vi "JSON to Variant.vi"(8 "error in (no error)":errorcluster, 10 "Variant (Data Type)":variant, 11 "JSON Value":refnum<class "JSON Value.lvclass">) -> (0 "error out":errorcluster, 2 "Variant out":variant)   [LabVIEW 2011, in "Variant JSON.lvlib"]
doc: "Converts a JSON value object into a LabVIEW datatype.\n\nElements in the <b>Variant (Data Type)</b> are used to retrieve information from <b>JSON Value</b>.\n\nCopyright 2012 James David Powell, Shaun Rumbell and Ton Plomp\nMore information on http://lavag.org/topic/16217-cr-json-labview"
uses:
  Variant JSON.lvlib
  JSON Value/JSON Value.lvclass
  JSON Object/JSON Object.lvclass
  JSON Value/Get as JSON string.vi
  JSON Scalar/Get as I32.vi
  JSON Scalar/Get as I64.vi
  JSON Scalar/Get as U32.vi
  JSON Scalar/Get as U64.vi
  JSON Scalar/Get as SGL.vi
  JSON Scalar/Get as DBL.vi
  JSON Scalar/Get as EXT.vi
  JSON Scalar/Get as Boolean.vi
  JSON Value/Get Item by name array.vi
  JSON Scalar/Get as Path.vi
  <userlib>/_OpenG.lib/array/array.llb/Conditional Auto-Indexing Tunnel (String)__ogtk.vi
  JSON Scalar/Get as Timestamp.vi
  JSON Scalar/JSON Scalar.lvclass
  Get Polymorphic/JSON GetSet.lvlib
  <vilib>/Utility/VariantDataType/VariantType.lvlib
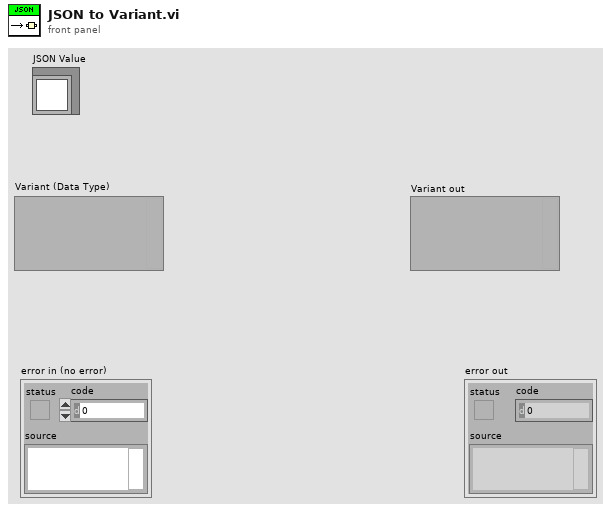
[diagram p1: front panel]
types:
  T1 = typedef "VariantType.lvlib/Type.ctl" = enum8{"Invalid Type", "Void", "I8", "I16", "I32", "I64", "U8", "U16", "U32", "U64", "Single Float", "Double Float", "Extended Float", "Single Complex", "Double Complex", "Extended Complex", "Enum U8", "Enum U16", "Enum U32", "Enum U64", "Single Float With Unit", "Double Float With Unit", "Extended Float With Unit", "Single Complex with Unit", "Double Complex with Unit", "Extended Complex with Unit", "Boolean", "String", "Path", "Picture", "Tag", "Array", "Cluster", "Variant", "LV Variant", "Waveform", "Timestamp", "Digital Waveform", "Digital Data", "ExpressData", "Refnum", "External Data", "VI", "Poly VI", "LabVIEW Class Instance", "Fixed Point"}
  T2 = typedef "JSON Scalar.lvclass/Variant Data Typdef.ctl" = cluster{"Type Enum":T1, "Name":string, "Variant":variant}
  T3 = cluster{"empty?":bool, "code":i32, "source":string}
  T4 = typedef "VariantType.lvlib/RefnumType.ctl" = enum16{"NotARefnum", "UnknownRefnum", "Generic", "Datalog", "ByteStream", "Device", "Occurence", "TCPNetConnection", "Auto", "Menu", "Imaq", "Hardware", "DataSocket", "Visa", "IVI", "UDPNetConnection", "Notifier", "Queue", "Irda", "EventReg", "DotNet", "UserEvent", "Callback", "UNUSED_EMPTY_POSITION", "BlueToothNetConnection", "LVObjApp", "LVObjVI", "LVObjUnknown", "GenericClass", "UserDefinedRefnumTag", "DataValue"}
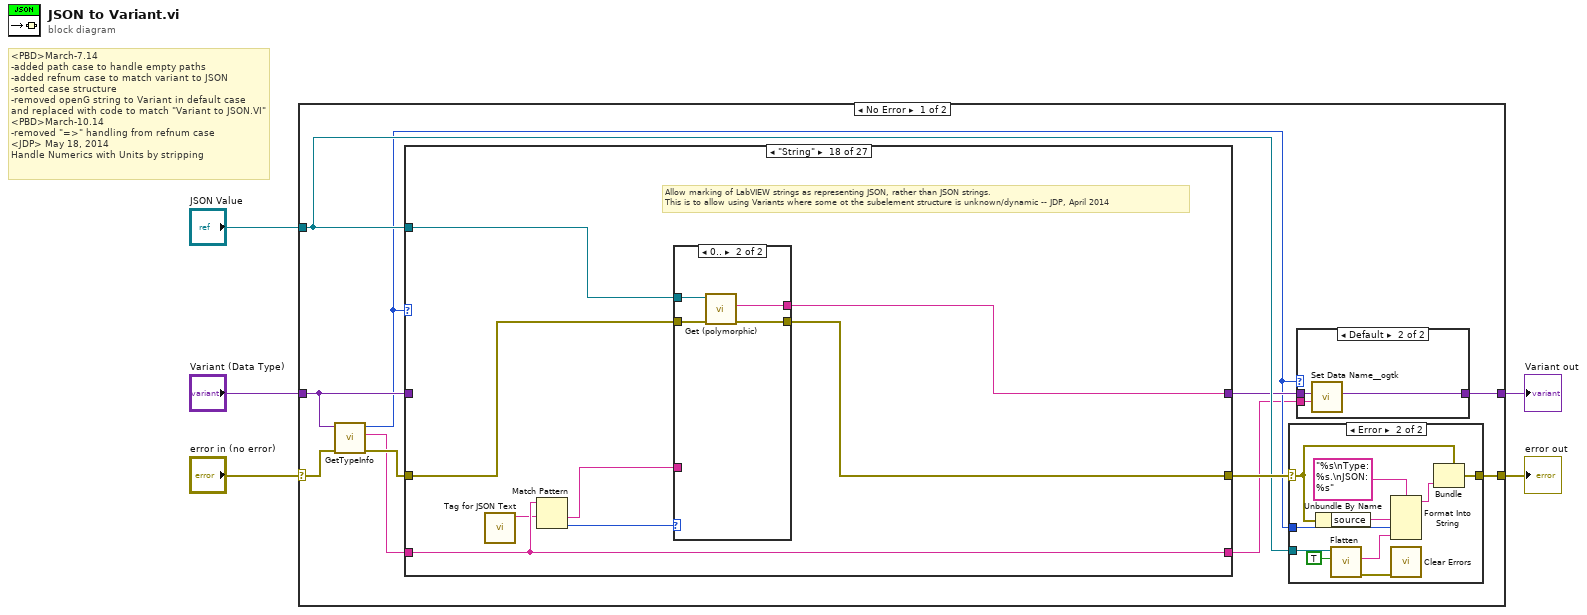
[diagram p0: block diagram]
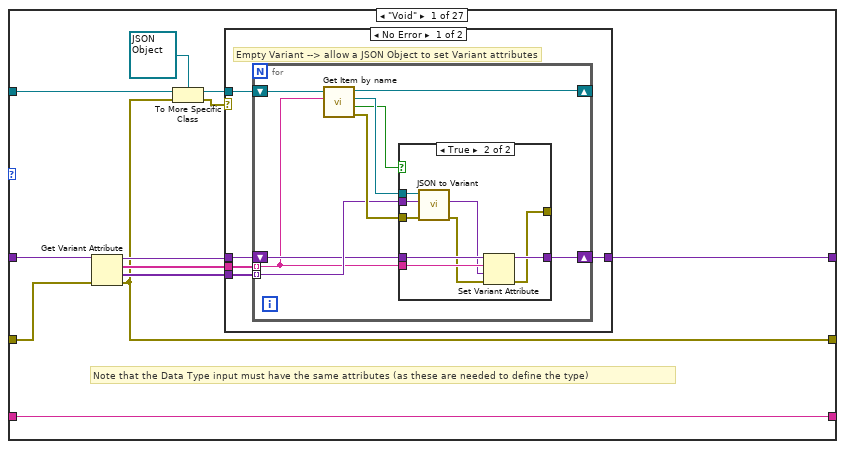
[diagram p4: hidden frame]
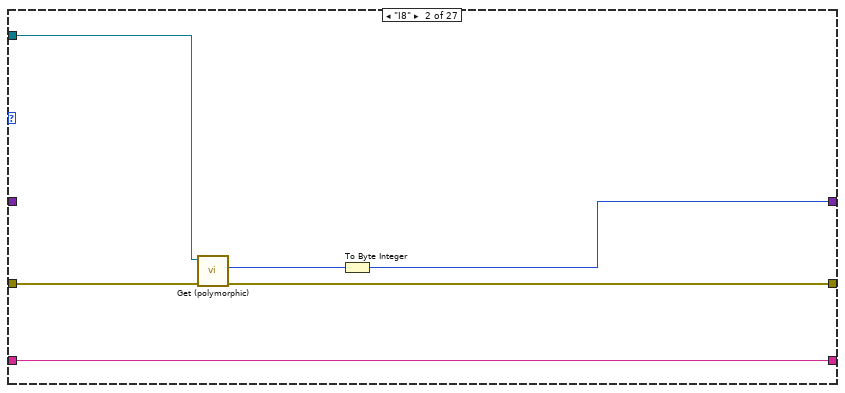
[diagram p7: hidden frame]
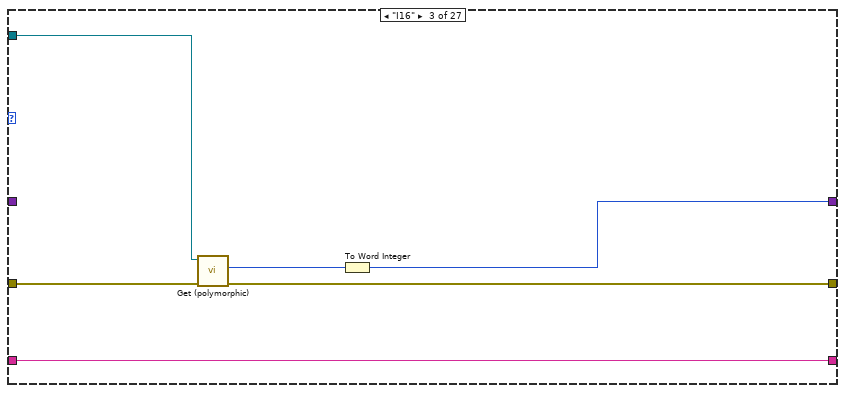
[diagram p8: hidden frame]
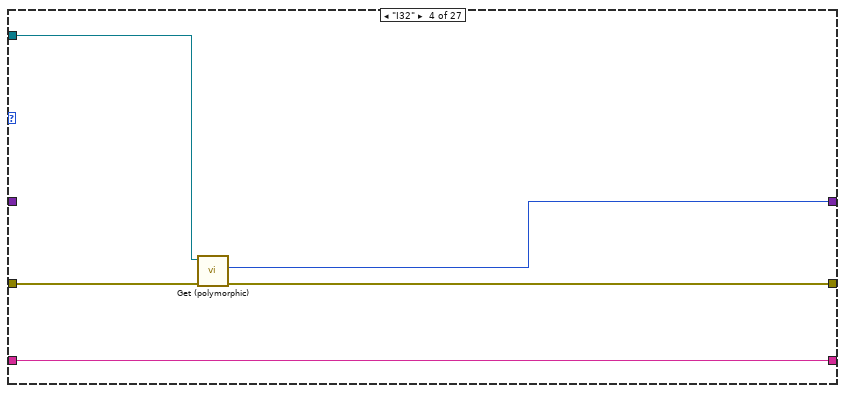
[diagram p9: hidden frame]
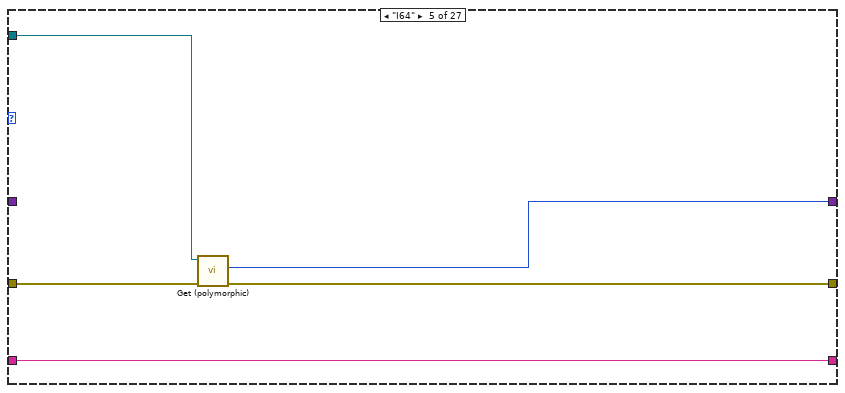
[diagram p10: hidden frame]
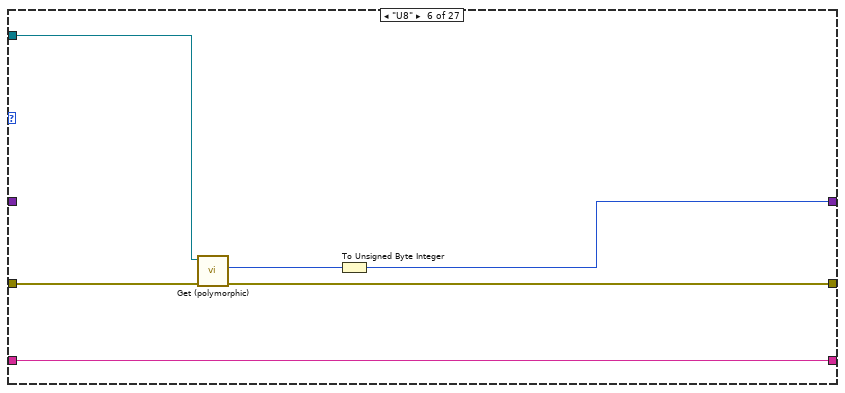
[diagram p11: hidden frame]
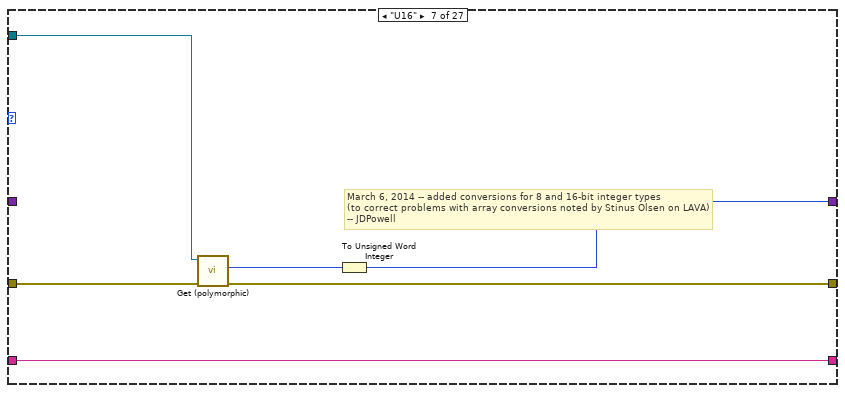
[diagram p12: hidden frame]
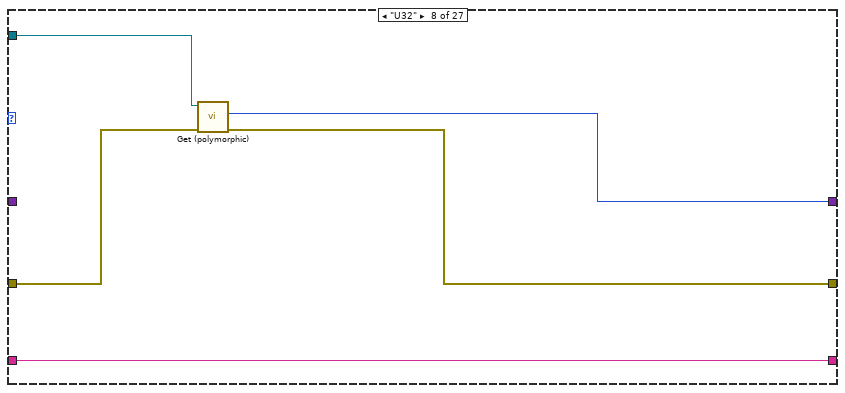
[diagram p13: hidden frame]
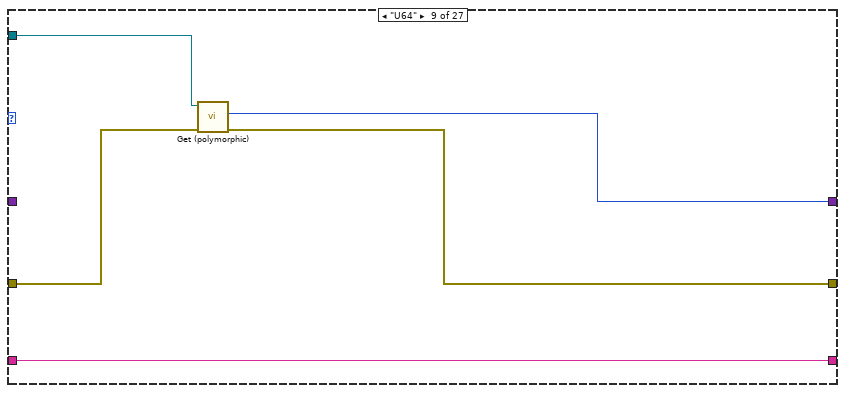
[diagram p14: hidden frame]
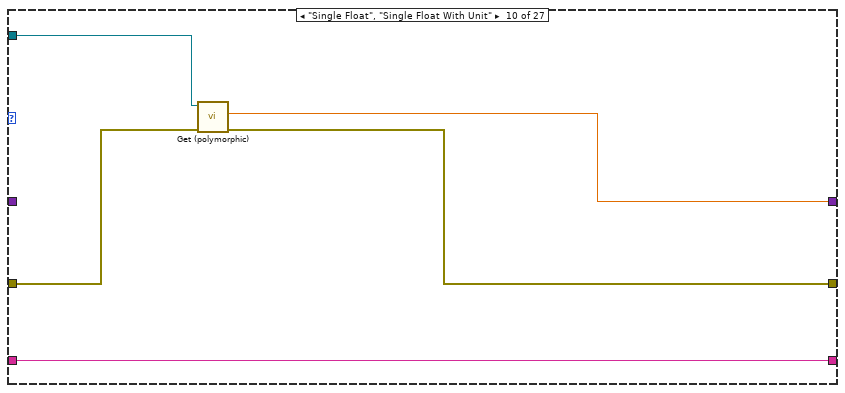
[diagram p15: hidden frame]
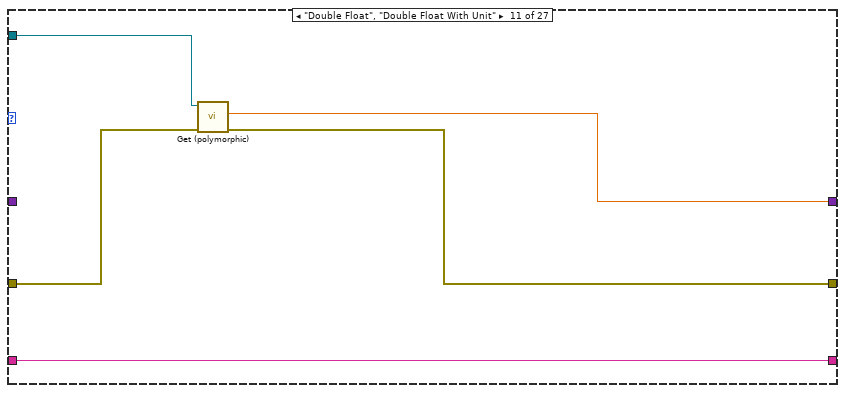
[diagram p16: hidden frame]
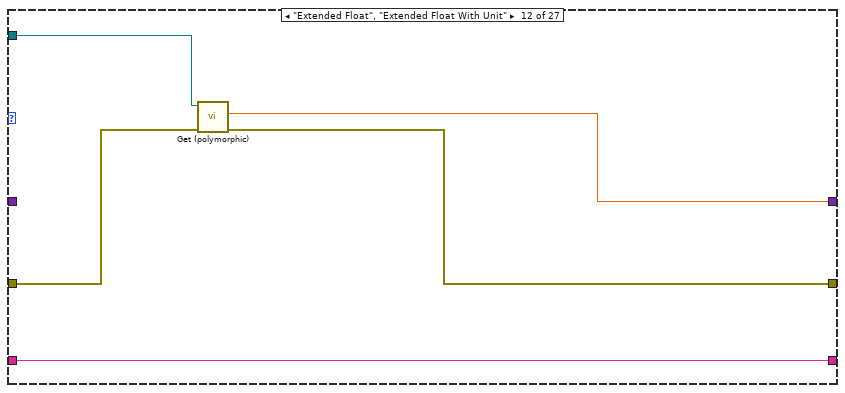
[diagram p17: hidden frame]
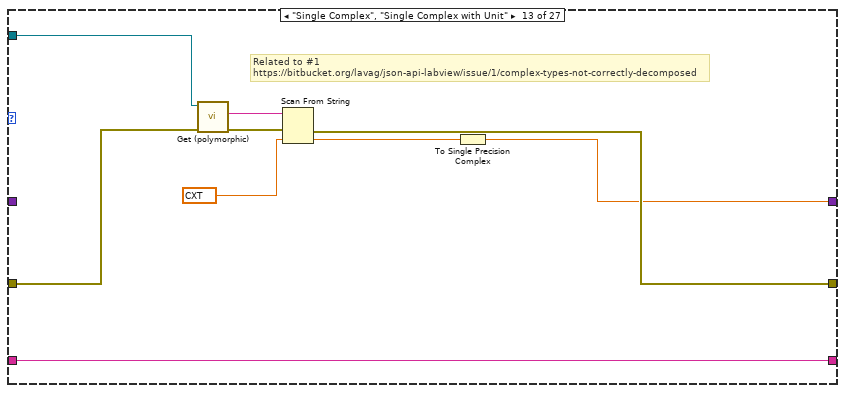
[diagram p18: hidden frame]
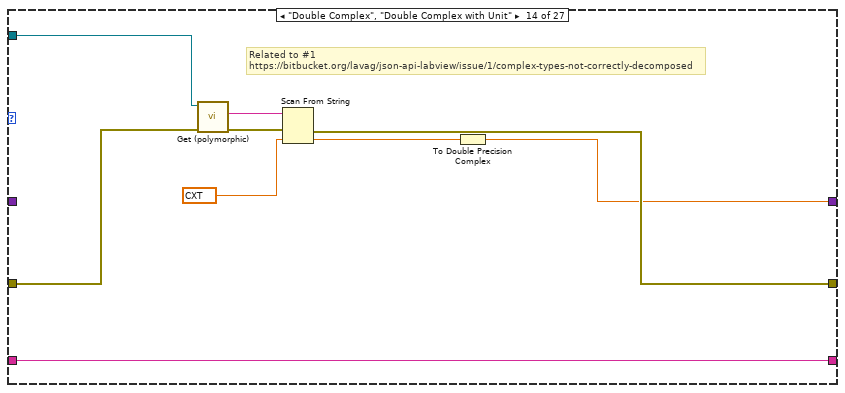
[diagram p19: hidden frame]
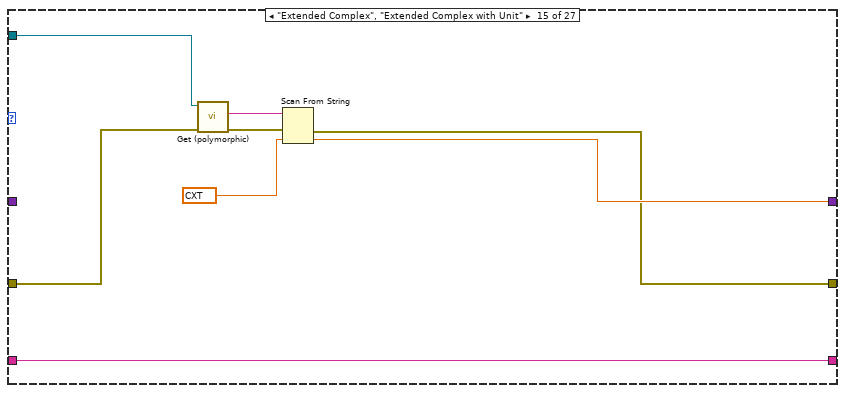
[diagram p20: hidden frame]
diagram:
  # "<PBD>March-7.14\n-added path case to handle empty paths\n-added refnum case to match variant to JSON\n-sorted case structure\n-removed openG string to Variant in default case \nand replaced with code to match \"Variant to JSON.VI\"\n<PBD>March-10.14\n-removed \"=>\" handling from refnum case\n<JDP> May 18, 2014\nHandle Numerics with Units by stripping"
  n1 = case shown="No Error" "error in (no error)" {
    selector: "error in (no error)" -> [w10 w326]
    tunnel: [w15 w326] -> w4
    tunnel: "Variant (Data Type)" -> [w11 w325]
    tunnel: "JSON Value" -> [w14 _]
    tunnel: [w12 w325] -> w1
    frame No Error {
      n2 = call <vilib>:"GetTypeInfo.vi"("error in (no error)"=w10, "Variant"=w11) -> ("error out"=w9:errorcluster, "Name"=w7:string, "Type Enum"=w8:T1)  [unwired: 5 in, 2 out]
      n3 = case shown="\"String\"" w8 {
        tunnel: w11 -> [w39 _ _ _ _ _ _ _ _ _ _ _ _ _ _ w162 _ _ _ w191 w199 w244 _ _ w262 w292 w321]
        tunnel: w9 -> [w34 w73 w79 w84 w89 w95 w101 w106 w111 w116 w121 w126 w136 w145 w153 w157 w165 w173 w187 w193 w198 w243 w249 w253 w261 _ w324]
        tunnel: [w33 w72 w78 w83 w88 w94 w100 w105 w110 w115 w120 w125 w131 w140 w148 w156 w164 w172 w186 w192 w205 w246 w248 w254 w258 w293 w319] -> w16
        tunnel: w14 -> [w43 w75 w81 w86 w91 w97 w103 w108 w113 w118 w123 w128 w137 w146 w154 w160 w167 w175 w188 w194 w203 w245 w251 w256 w260 w295 w323]
        tunnel: [w35 w71 w77 w85 w90 w93 w99 w107 w112 w117 w122 w127 w130 w139 w150 w161 w166 w174 w185 w189 w201 w238 w250 w255 w259 w294 w318] -> w13
        tunnel: w7 -> [w32 w70 w76 w82 w87 w92 w98 w104 w109 w114 w119 w124 w129 w138 w147 w155 w163 w171 w184 w190 w195 w237 w247 w252 w257 w301 w316]
        tunnel: [w32 w70 w76 w82 w87 w92 w98 w104 w109 w114 w119 w124 w129 w138 w147 w155 w163 w171 w184 w190 w195 w237 w247 w252 w257 w301 w316] -> w6
        frame "Void" {
          # "Note that the Data Type input must have the same attributes (as these are needed to define the type)"
          n4 = Get Variant Attribute(Variant=w39, error in=w34) -> (duplicate Variant=w38:variant, names=w37:string[], values=w36:variant[], error out=w33:errorcluster)  [unwired: 2 in]
          n5 = To More Specific Class(target class=refnum<class "JSON Object.lvclass"> refnum ("JSON Object in"), reference=w43, error in=w33) -> (specific class reference=w41:refnum<class "JSON Object.lvclass">, error out=w40:errorcluster)
          n6 = case shown="No Error" w40 {
            tunnel: w41 -> [w45 _]
            tunnel: w38 -> [w46 w69]
            tunnel: w37 -> [w48 _]
            tunnel: w36 -> [w47 _]
            tunnel: [w44 w69] -> w35
            frame No Error {
              # "Empty Variant --> allow a JSON Object to set Variant attributes"
              n7 = for {
                tunnel: w48 -> [w51] mode=indexing
                tunnel: w47 -> [w53] mode=indexing
                shift-right: [w50] -> w44
                shift-left: w46 -> [w52]
                shift-right: [w49] -> _
                shift-left: w45 -> [w54]
                n8 = call-dynamic "Get Item by name.vi"("name"=w51, "JSON Object in"=w54) -> ("error out"=w57:errorcluster, "found"=w55:bool, "Value"=w56:refnum<class "JSON Value.lvclass">, "JSON Object out"=w49:refnum<class "JSON Object.lvclass">)  [unwired: 6 in]
                n9 = case shown="True" w55 {
                  tunnel: w57 -> [w59 w68]
                  tunnel: [w59 w60] -> _
                  tunnel: w53 -> [_ w67]
                  tunnel: w56 -> [_ w66]
                  tunnel: w52 -> [w58 w65]
                  tunnel: w51 -> [_ w64]
                  tunnel: [w58 w63] -> w50
                  frame False {
                  }
                  frame True {
                    n10 = call "JSON to Variant.vi"("error in (no error)"=w68, "Variant (Data Type)"=w67, "JSON Value"=w66) -> ("error out"=w61:errorcluster, "Variant out"=w62:variant)  [unwired: 7 in]
                    n11 = Set Variant Attribute(Variant=w65, name=w64, value=w62, error in=w61) -> (Variant out=w63:variant, error out=w60:errorcluster)  [unwired: 1 out]
                  }
                }
              }
            }
            frame Error {
            }
          }
        }
        frame "I8" {
          n12 = call-poly "Get (polymorphic).vi"("error in (no error)"=w73, "JSON Scalar in"=w75) -> ("error out"=w72:errorcluster, "Number"=w74:i32)  [unwired: 7 in, 1 out]
          n13 = To Byte Integer(number=w74) -> (8bit integer=w71:i8)
        }
        frame "I16" {
          n14 = call-poly "Get (polymorphic).vi"("error in (no error)"=w79, "JSON Scalar in"=w81) -> ("error out"=w78:errorcluster, "Number"=w80:i32)  [unwired: 7 in, 1 out]
          n15 = To Word Integer(number=w80) -> (16bit integer=w77:i16)
        }
        frame "I32" {
          n16 = call-poly "Get (polymorphic).vi"("error in (no error)"=w84, "JSON Scalar in"=w86) -> ("error out"=w83:errorcluster, "Number"=w85:i32)  [unwired: 7 in, 1 out]
        }
        frame "I64" {
          n17 = call-poly "Get (polymorphic).vi"("error in (no error)"=w89, "JSON Scalar in"=w91) -> ("error out"=w88:errorcluster, "Number"=w90:i64)  [unwired: 7 in, 1 out]
        }
        frame "U8" {
          n18 = call-poly "Get (polymorphic).vi"("error in (no error)"=w95, "JSON Scalar in"=w97) -> ("error out"=w94:errorcluster, "Number"=w96:u32)  [unwired: 7 in, 1 out]
          n19 = To Unsigned Byte Integer(number=w96) -> (unsigned 8bit integer=w93:u8)
        }
        frame "U16" {
          # "March 6, 2014 -- added conversions for 8 and 16-bit integer types\n(to correct problems with array conversions noted by Stinus Olsen on LAVA)\n-- JDPowell"
          n20 = call-poly "Get (polymorphic).vi"("error in (no error)"=w101, "JSON Scalar in"=w103) -> ("error out"=w100:errorcluster, "Number"=w102:u32)  [unwired: 7 in, 1 out]
          n21 = To Unsigned Word Integer(number=w102) -> (unsigned 16bit integer=w99:u16)
        }
        frame "U32" {
          n22 = call-poly "Get (polymorphic).vi"("error in (no error)"=w106, "JSON Scalar in"=w108) -> ("error out"=w105:errorcluster, "Number"=w107:u32)  [unwired: 7 in, 1 out]
        }
        frame "U64" {
          n23 = call-poly "Get (polymorphic).vi"("error in (no error)"=w111, "JSON Scalar in"=w113) -> ("error out"=w110:errorcluster, "Number"=w112:u64)  [unwired: 7 in, 1 out]
        }
        frame "Single Float", "Single Float With Unit" {
          n24 = call-poly "Get (polymorphic).vi"("error in (no error)"=w116, "JSON Value in"=w118) -> ("error out"=w115:errorcluster, "Number"=w117:sgl)  [unwired: 7 in, 1 out]
        }
        frame "Double Float", "Double Float With Unit" {
          n25 = call-poly "Get (polymorphic).vi"("error in (no error)"=w121, "JSON Value in"=w123) -> ("error out"=w120:errorcluster, "Number"=w122:dbl)  [unwired: 7 in, 1 out]
        }
        frame "Extended Float", "Extended Float With Unit" {
          n26 = call-poly "Get (polymorphic).vi"("error in (no error)"=w126, "JSON Value in"=w128) -> ("error out"=w125:errorcluster, "Number"=w127:ext)  [unwired: 7 in, 1 out]
        }
        frame "Single Complex", "Single Complex with Unit" {
          # "Related to #1\nhttps://bitbucket.org/lavag/json-api-labview/issue/1/complex-types-not-correctly-decomposed"
          n27 = call-poly "Get (polymorphic).vi"("error in (no error)"=w136, "JSON Scalar in"=w137) -> ("error out"=w132:errorcluster, "LabVIEW Text"=w135:string)  [unwired: 7 in, 1 out]
          n28 = Scan From String(input string=w135, error in=w132, default 1=cxt 0.0+0.0i) -> (error out=w131:errorcluster, output 1=w133:cxt)  [unwired: 2 in, 2 out]
          n29 = To Single Precision Complex(1:w133) -> (0:w130:csg)
        }
        frame "Double Complex", "Double Complex with Unit" {
          # "Related to #1\nhttps://bitbucket.org/lavag/json-api-labview/issue/1/complex-types-not-correctly-decomposed"
          n30 = call-poly "Get (polymorphic).vi"("error in (no error)"=w145, "JSON Scalar in"=w146) -> ("error out"=w141:errorcluster, "LabVIEW Text"=w144:string)  [unwired: 7 in, 1 out]
          n31 = Scan From String(input string=w144, error in=w141, default 1=cxt 0.0+0.0i) -> (error out=w140:errorcluster, output 1=w142:cxt)  [unwired: 2 in, 2 out]
          n32 = To Double Precision Complex(1:w142) -> (0:w139:cdb)
        }
        frame "Extended Complex", "Extended Complex with Unit" {
          n33 = call-poly "Get (polymorphic).vi"("error in (no error)"=w153, "JSON Scalar in"=w154) -> ("error out"=w149:errorcluster, "LabVIEW Text"=w152:string)  [unwired: 7 in, 1 out]
          n34 = Scan From String(input string=w152, error in=w149, default 1=cxt 0.0+0.0i) -> (error out=w148:errorcluster, output 1=w150:cxt)  [unwired: 2 in, 2 out]
        }
        frame "Enum U8".."Enum U64" {
          n35 = call-poly "Get (polymorphic).vi"("error in (no error)"=w157, "JSON Scalar in"=w160) -> ("error out"=w158:errorcluster, "LabVIEW Text"=w159:string)  [unwired: 7 in, 1 out]
          n36 = call <userlib>:"Set Enum String Value__ogtk.vi"("error in (no error)"=w158, "String Value"=w159, "Default Enum Value"=w162) -> ("error out"=w156:errorcluster, "Enum"=w161:variant)  [unwired: 7 in]
        }
        frame "Boolean" {
          n37 = call-poly "Get (polymorphic).vi"("error in (no error)"=w165, "JSON Value in"=w167) -> ("error out"=w164:errorcluster, "Boolean"=w166:bool)  [unwired: 7 in, 1 out]
        }
        frame "String" {
          # "Allow marking of LabVIEW strings as representing JSON, rather than JSON strings.\nThis is to allow using Variants where some ot the subelement structure is unknown/dynamic -- JDP, April 2014"
          n38 = call "Tag for JSON Text.vi"() -> ("Tag for JSON text"=w168:string)  [unwired: 11 in]
          n39 = Match Pattern(string=w171, regular expression=w168) -> (after substring=w170:string, offset past match=w169:i32)  [unwired: 1 in, 2 out]
          n40 = case shown="0.." w169 {
            tunnel: w175 -> [w179 w183]
            tunnel: [w178 w182] -> w174
            tunnel: w173 -> [w177 w181]
            tunnel: [w176 w180] -> w172
            tunnel: w170 -> [_ _]
            frame ..-1 {
              n41 = call-poly "Get (polymorphic).vi"("error in (no error)"=w177, "JSON Scalar in"=w179) -> ("error out"=w176:errorcluster, "LabVIEW Text"=w178:string)  [unwired: 7 in, 1 out]
            }
            frame 0.. {
              n42 = call-poly "Get (polymorphic).vi"("error in (no error)"=w181, "JSON Value in"=w183) -> ("error out"=w180:errorcluster, "String"=w182:string)  [unwired: 8 in]
            }
          }
        }
        frame "Path" {
          n43 = call-poly "Get (polymorphic).vi"("error in (no error)"=w187, "JSON Scalar in"=w188) -> ("error out"=w186:errorcluster, "path"=w185:path)  [unwired: 7 in, 1 out]
        }
        frame "Array" {
          # "Dec 2015, JDP rewrite for higher speed with large arrays"
          n44 = call "Get Array as Variant.vi"("error in (no error)"=w193, "Variant (Data Type)"=w191, "JSON Value in"=w194) -> ("error out"=w192:errorcluster, "Default VData"=w189:variant)  [unwired: 7 in]
        }
        frame "Cluster" {
          w204 = 91 items=["No error", "Argument error", "Memory is full", "Out of zone", "End of file", "File already open", "Generic file I/O error", "File not found", "File permission error", "Disk is full", "Duplicate path", "Too many files open", "System feature not enabled", "Resource file not found", "Cannot add resource", "Resource not found", "Image not found", "Image memory error", "Pen does not exist", "Config type invalid", "Config token not found", "Config parse error", "Config memory error", "Bad external code format", "Bad external code offset", "External code not present", "Null window", "Destroy window error", "Null menu", "Print aborted", "Bad print record", "Print driver error", "Windows error during printing", "Memory error during printing", "Print dialog error", "Generic print error", "Invalid device refnum", "Device not found", "Device parameter error", "Device unit error", "Cannot open device", "Device call aborted", "Generic error", "Cancelled by user", "Object ID too low", "Object ID too high", "Object not in heap", "Unknown heap", "Unknown object (invalid DefProc)", "Unknown object (DefProc not in table)", "Message out of range", "Invalid (null) method", "Unknown message", "Manager call not supported", "Bad address", "Network operation in progress", "Network operation timed out", "Connection is busy", "Network attribute not supported", "Network error", "Address in use", "System out of memory", "Connection aborted", "Connection refused", "Not connected", "Already connected", "Connection closed", "Initialization error (interapplication manager)", "Bad occurrence", "Wait on unbound occurrence handler", "Occurrence queue overflow", "Datalog type conflict", "Unused", "Unrecognized type (interapplication manager)", "Memory corrupt", "Failed to make temporary DLL", "Old CIN version", "Drag socket not found", "Failed to load drop-object", "Failed to register OLE object", "Failed to release OLE object", "Format specifier type mismatch", "Unknown format specifier", "Too few format specifiers", "Too many format specifiers", "Scan failed", "Newer CIN version", "Error converting to variant", "Runtime menu error", "Password tampered", "Variant attribute not found", "Incompatible variant data type", "Event data is not available", "Event Store is not present", "Occurrence is not found", "Event Queue is not created", "Event info is not available", "Refnum passed is NULL", "Error retrieving Class GUID", "Error retrieving CoClass GUID", "Error retrieving TypeLib GUID.", "Bad built application magic bytes.", "Specific driver is different from the specific driver associated with the Logical Name.", "There is no session opened to the class driver.", "Max Error", "MAX - Error with config objects", "MAX - Error loading configuration", "MAX - Group not supported"]
          # "If an elements fails, set a warning (91)\nIncluding the source JSON string."
          # "<ToDo>\nGo over this error logic"
          # "Throw warning,\nnot an error."
          n45 = call "Variant Decode.vi"("error in (no error)"=w198, "variant"=w199) -> ("error out"=w196:errorcluster, "Variant Data"=w197:T2[])  [unwired: 7 in, 1 out]
          n46 = for {
            shift-right: [w228] -> _
            shift-left: w203 -> [w229]
            tunnel: [w225] -> w202 mode=indexing
            tunnel: [w227] -> w217 mode=indexing
            tunnel: [w221] -> w216 mode=indexing
            tunnel: w197 -> [w224] mode=indexing
            n47 = call "Handle JSON Text Tag.vi"("Variant Data"=w224) -> ("Variant Data (tag stripped)"=w223:T2)  [unwired: 9 in, 1 out]
            n48 = Unbundle By Name(w223) -> ("Name"=w221:string, "Variant"=w222:variant)
            n49 = call-dynamic "Get Item by name.vi"("name"=w221, "JSON Value In"=w229) -> ("error out"=w220:errorcluster, "found"=w218:bool, "Value"=w219:refnum<class "JSON Value.lvclass">, "JSON Value Out"=w228:refnum<class "JSON Value.lvclass">)  [unwired: 6 in]
            n50 = case shown="True" w218 {
              tunnel: w220 -> [w230 w236]
              tunnel: [w230 w235] -> w226
              tunnel: w222 -> [w231 w234]
              tunnel: w219 -> [_ w233]
              tunnel: [w231 w232] -> w225
              frame False {
              }
              frame True {
                n51 = call "JSON to Variant.vi"("error in (no error)"=w236, "Variant (Data Type)"=w234, "JSON Value"=w233) -> ("error out"=w235:errorcluster, "Variant out"=w232:variant)  [unwired: 7 in]
              }
            }
            n52 = Unbundle By Name(w226) -> ("status"=w227:bool)
          }
          n53 = call <userlib>:"Array of VData to VCluster__ogtk.vi"("error in (no error)"=w196, "Array"=w202) -> ("error out"=w200:errorcluster, "VCluster"=w201:variant)  [unwired: 8 in]
          n54 = call-poly <userlib>:"Conditional Auto-Indexing Tunnel__ogtk.vi"("Array in"=w216, "Elements to keep"=w217) -> ("Filtered Array out"=w211:string[])  [unwired: 5 in]
          n55 = Array To Spreadsheet String(delimiter (Tab)="\r\n", array=w211, 3:"%s" ("format string")) -> (spreadsheet string=w212:string)
          n56 = Empty Array?(array=w211) -> (empty?=w208:bool)
          n57 = Format Into String(format string="Failed elements:\n%s", w212) -> (resulting string=w207:string)  [unwired: 2 in, 1 out]
          n58 = Bundle("empty?"=w208, w204, w207) -> (w209:cluster{"empty?":bool, i32, string})  [unwired: 1 in]
          n59 = Select(t=errorcluster {"status"=FALSE, "code"=0, "source"=""} ("error out"), s=w208, f=w209) -> (s? t:f=w206:T3)
          n60 = Merge Errors(w200, w206) -> (w205:errorcluster)
        }
        frame "Variant", "LV Variant" {
          # "Get item inside variant, convert, and then put back in a variant"
          n61 = Variant To Data(error in=w243, type=variant, Variant=w244) -> (data=w241:variant, error out=w242:errorcluster)
          n62 = call "JSON to Variant.vi"("error in (no error)"=w242, "Variant (Data Type)"=w241, "JSON Value"=w245) -> ("error out"=w246:errorcluster, "Variant out"=w239:variant)  [unwired: 7 in]
          n63 = To Variant(anything=w239) -> (Variant=w238:variant)
        }
        frame "Waveform" {
          n64 = call "Get as Waveform.vi"("error in (no error)"=w249, "JSON Value In"=w251) -> ("error out"=w248:errorcluster, "Waveform"=w250:waveform(dbl))  [unwired: 7 in, 1 out]
        }
        frame "Timestamp" {
          n65 = call-poly "Get (polymorphic).vi"("error in (no error)"=w253, "JSON Value in"=w256) -> ("error out"=w254:errorcluster, "Time Stamp"=w255:timestamp)  [unwired: 7 in, 1 out]
        }
        frame "Refnum" {
          n66 = call-poly "Get (polymorphic).vi"("error in (no error)"=w261, "JSON Scalar in"=w260) -> ("error out"=w264:errorcluster, "LabVIEW Text"=w263:string)  [unwired: 7 in, 1 out]
          n67 = call <vilib>:"GetRefnumInfo.vi"("error in (no error)"=w264, "Variant"=w262) -> ("error out"=w265:errorcluster, "ReferenceType"=w266:T4)  [unwired: 6 in, 2 out]
          n68 = case shown="\"Visa\", \"IVI\", \"UserDefinedRefnumTag\"" w266 {
            tunnel: [w267 w276 w289] -> w259
            tunnel: w265 -> [w268 w270 w287]
            tunnel: [w268 w269 w288] -> w258
            tunnel: w263 -> [_ w271 w284]
            tunnel: w262 -> [w267 w279 w291]
            frame "NotARefnum", "UnknownRefnum" {
            }
            frame "Visa", "IVI", "UserDefinedRefnumTag" {
              n69 = Variant To Data(error in=w270, type="", Variant=w279) -> (data=w277:string, error out=w269:errorcluster)
              n70 = Scan From String(input string=w271, default 1=w277) -> (error out=w275:errorcluster, output 1=w272:string)  [unwired: 3 in, 2 out]
              n71 = Select(t="", s=w275, f=w272) -> (s? t:f=w274:string)
              n72 = To Variant(anything=w274) -> (Variant=w276:variant)
            }
            frame Default {
              w283 = 0
              n73 = Scan From String(input string=w284, default 1=w283) -> (error out=w286:errorcluster, output 1=w285:i32)  [unwired: 3 in, 2 out]
              n74 = Select(t=w283, s=w286, f=w285) -> (s? t:f=w281:i32)
              n75 = Variant To Flattened String(Variant=w291) -> (1:w290:i16[])  [unwired: 1 out]
              n76 = Type Cast(type="", x=w281) -> (*(type *) &x=w282:string)
              n77 = Flattened String To Variant(4:w287, 6:w282, 7:w290) -> (0:w288:errorcluster, 3:w289:variant)
            }
          }
        }
        frame "LabVIEW Class Instance" {
          w296 = refnum<class "JSON Value.lvclass"> refnum ("JSON Value")
          n78 = Variant To Data(type=refnum<class> refnum ("LabVIEW Object"), Variant=w292) -> (data=w297:refnum<class>, error out=w299:errorcluster)  [unwired: 1 in]
          n79 = To More Specific Class(target class=w296, reference=w297, error in=w299) -> (error out=w298:errorcluster)  [unwired: 1 out]
          n80 = case shown="No Error" w298 {
            selector: w298 -> [w309 _]
            tunnel: w297 -> [w308 _]
            tunnel: w296 -> [w307 _]
            tunnel: w295 -> [w303 w315]
            tunnel: [w306 w312] -> w294
            tunnel: [w305 w313] -> w293
            tunnel: w292 -> [_ w311]
            frame No Error {
              # "Needed to get the wire type of the \nVariant to be the right subclass"
              # "Target is a JSON Value (or subclass), so"
              n81 = To More Specific Class(target class=w307, reference=w308, error in=w309) -> (specific class reference=w302:refnum<class "JSON Value.lvclass">, error out=w304:errorcluster)
              n82 = call-dynamic "Place in Variant.vi"("error in (no error)"=w304, "object"=w303, "wire type"=w302) -> ("error out"=w305:errorcluster, "variant (of wire type, containing object)"=w306:variant)  [unwired: 7 in]
            }
            frame Error {
              # "Fixed 3-Sep-2015 -- JDP"
              # "Try and unflatten to the supplied datatype"
              n83 = call "Get as Text.vi"("JSON Scalar in"=w315) -> ("LabVIEW Text"=w314:string)  [unwired: 8 in, 2 out]
              n84 = Variant To Flattened String(Variant=w311) -> (1:w310:i16[])  [unwired: 1 out]
              n85 = Flattened String To Variant(6:w314, 7:w310) -> (0:w313:errorcluster, 3:w312:variant)  [unwired: 1 in]
            }
          }
        }
        frame Default {
          # "Try and unflatten to the supplied data type"
          n86 = call "Get as Text.vi"("error in (no error)"=w324, "JSON Scalar in"=w323) -> ("error out"=w320:errorcluster, "LabVIEW Text"=w317:string)  [unwired: 7 in, 1 out]
          n87 = Variant To Flattened String(Variant=w321) -> (1:w322:i16[])  [unwired: 1 out]
          n88 = Flattened String To Variant(4:w320, 6:w317, 7:w322) -> (0:w319:errorcluster, 3:w318:variant)
        }
      }
      n89 = case shown="Error" w16 {
        selector: w16 -> [w21 w26]
        tunnel: [w21 w24] -> w15
        tunnel: w8 -> [_ w29]
        tunnel: w14 -> [_ w28]
        frame No Error {
        }
        frame Error {
          n90 = Unbundle By Name(w26) -> ("source"=w31:string)
          n91 = call-dynamic "Flatten.vi"("Pretty Print?"=TRUE, "JSON Value in"=w28) -> ("error out"=w23:errorcluster, "String"=w27:string)  [unwired: 8 in]
          n92 = Format Into String(format string="%s\nType: %s.\nJSON: %s", w31, w29, w27) -> (resulting string=w25:string)  [unwired: 2 in, 1 out]
          n93 = call <vilib>:"Clear Errors.vi"("error in (no error)"=w23) -> ()  [unwired: 6 in, 1 out]
          n94 = Bundle(cluster=w26, "source"=w25) -> (w24:errorcluster)  [unwired: 2 in]
        }
      }
      n95 = case shown="Default" w8 {
        tunnel: w13 -> [w17 w20]
        tunnel: [w17 w19] -> w12
        tunnel: w6 -> [_ w18]
        frame "Void" {
          # "needed because\nSet Data Name will \nerror out and clear\nattributes for Void type"
        }
        frame Default {
          n96 = call <userlib>:"Set Data Name__ogtk.vi"("Data Name"=w18, "Data"=w20) -> ("Renamed Data"=w19:variant)  [unwired: 8 in, 1 out]
        }
      }
    }
    frame Error {
    }
  }
  "error out" <- w4
  "Variant out" <- w1
